vi "Flash FPGA.vi"(8 "Error In":errorcluster, 10 "Bit File Path":path, 11 "Adept Config":T1) -> (0 "Error Out":errorcluster, 2 "Success?":bool, 3 "Adept Config":T1)   [LabVIEW 2011, in "LVH-Adept.lvlib"]
doc: "Flash a bitfile to a Digilent FPGA board."
uses:
  LVH-Adept.lvlib
  Private/Type Defs/Device Config.ctl
  Private/Type Defs/Status.ctl
  Private/DJTG/DJTG.lvlib
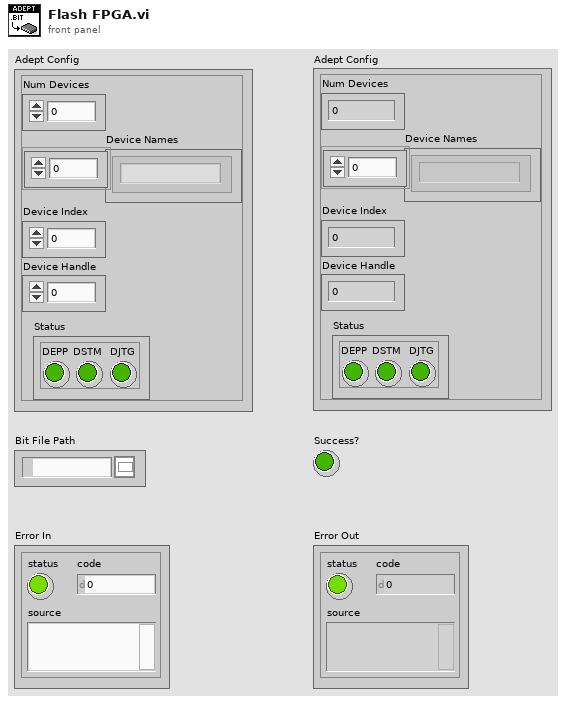
[diagram p1: front panel]
types:
  T1 = typedef "LVH-Adept.lvlib/Device Config.ctl" = cluster{"Num Devices":i32, "Device Names":string[], "Device Index":u16, "Device Handle":u32, "Status":T2}
  T2 = typedef "LVH-Adept.lvlib/Status.ctl" = cluster{"DEPP":bool, "DSTM":bool, "DJTG":bool}
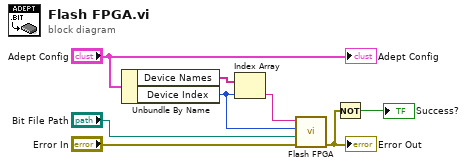
[diagram p0: block diagram]
diagram:
  n1 = Unbundle By Name("Adept Config") -> ("Device Names"=w8:string[], "Device Index"=w6:u16)
  n2 = Index Array(array=w8, index=w6) -> (element=w7:string)
  n3 = call "Flash FPGA.vi"("Error In"="Error In", "Bit File Path"="Bit File Path", "Device ID"=w6, "Device Name"=w7) -> ("Error Out"=w1:errorcluster)  [unwired: 7 in]
  "Error Out" <- w1
  n4 = Not(x=w1) -> (.not. x?=→"Success?":bool)
  "Adept Config" <- "Adept Config"
